vi "Scan Distributed Nodes.vi"(6 "ScanPeroid(>2000ms)":u32=2000, 8 "error in (no error)":errorcluster, 11 "Report Address":cluster{"address":string, "receiver port":u16}={"address"="234.5.6.7", "receiver port"=58432}) -> (0 "error out":errorcluster, 3 "Information":T1(array[cluster]))   [LabVIEW 2017]
doc: "Creates a read-only UDP multicast session and receives data on the specified port."
uses:
  _Typedef/Def-Report -- Cluster.ctl
  <vilib>/Utility/tcp.llb/UDP Multicast Read-Only Open.vi
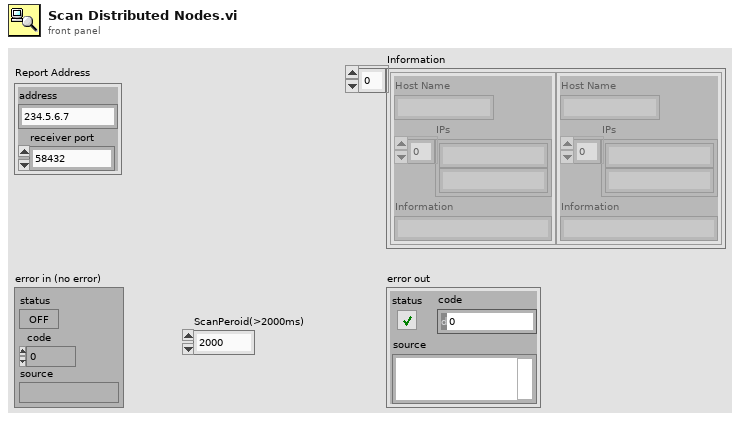
[diagram p1: front panel]
types:
  T1 = cluster{"Host Name":string, "IPs":string[], "Information":string}[]
  T2 = typedef "Def-Report -- Cluster.ctl" = cluster{"Host Name":string, "IPs":string[], "Timestamp":string, "Information":string}
  T3 = cluster{"Host Name":string, "IPs":string[], "Information":string}
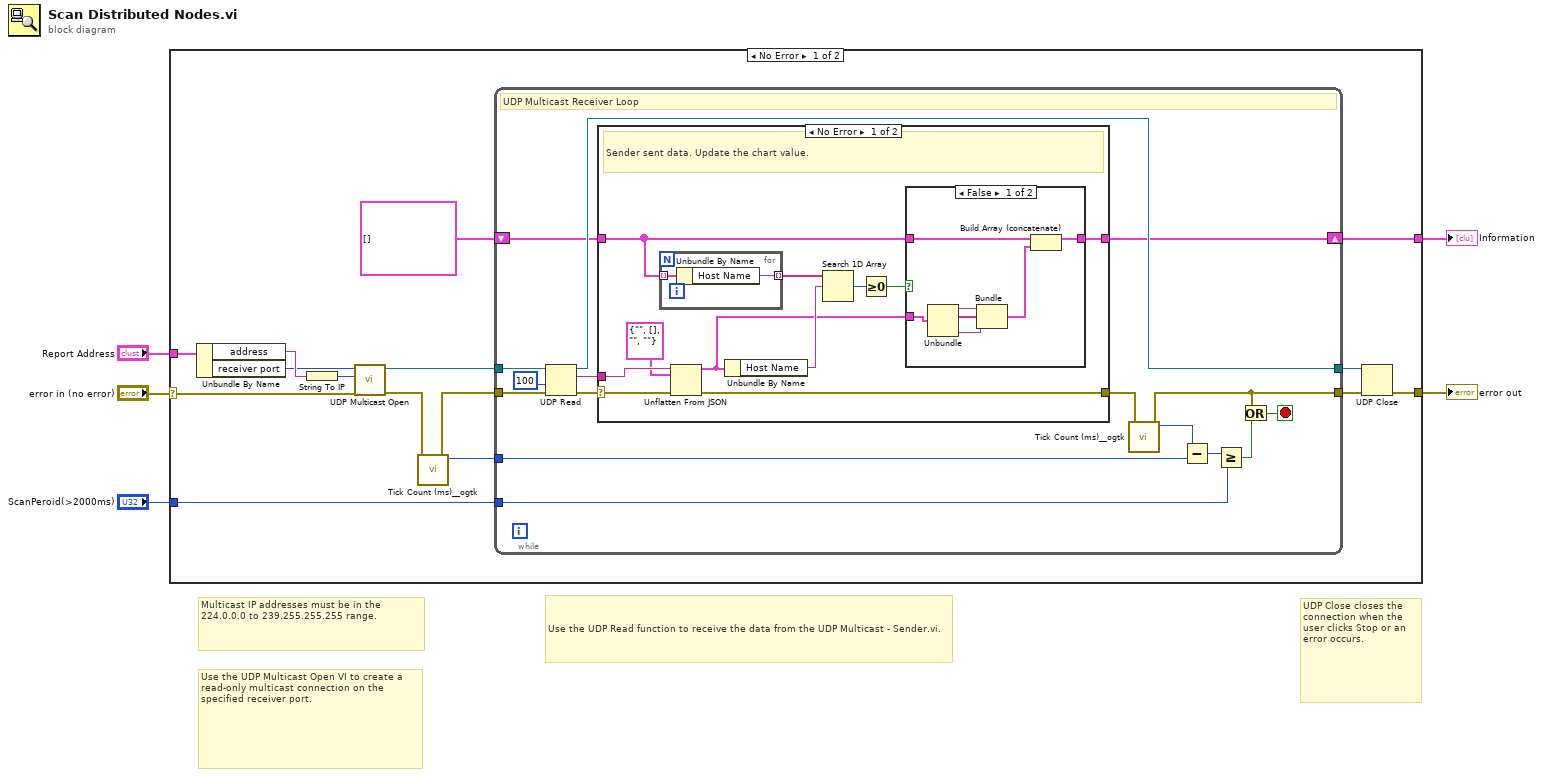
[diagram p0: block diagram]
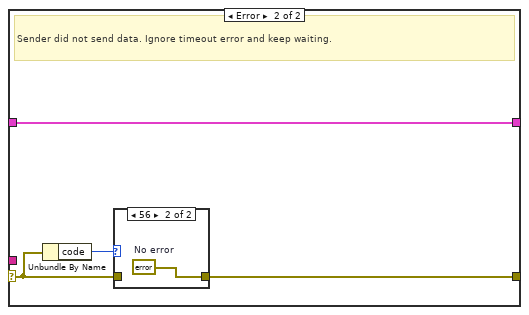
[diagram p3: hidden frame]
diagram:
  # "UDP Close closes the connection when the user clicks Stop or an error occurs."
  # "Use the UDP Multicast Open VI to create a read-only multicast connection on the specified receiver port."
  # "Multicast IP addresses must be in the 224.0.0.0 to 239.255.255.255 range."
  # "Use the UDP Read function to receive the data from the UDP Multicast - Sender.vi."
  n1 = case shown="No Error" "error in (no error)" {
    selector: "error in (no error)" -> [w12 w64]
    tunnel: "Report Address" -> [w15 _]
    tunnel: [w11 w64] -> w3
    tunnel: "ScanPeroid(>2000ms)" -> [w8 _]
    tunnel: [w6 _] -> w1
    frame No Error {
      n2 = Unbundle By Name(w15) -> ("address"=w14:string, "receiver port"=w13:u16)
      n3 = String To IP(1:w14) -> (0:w16:u32)
      n4 = call-poly <vilib>:"UDP Multicast Open.vi"("error in (no error)"=w12, "multicast addr"=w16, "port"=w13) -> ("error out"=w18:errorcluster, "connection ID"=w17:refnum<k16>)  [unwired: 6 in, 1 out]
      n5 = call <userlib>:"Tick Count (ms)__ogtk.vi"("error in (no error)"=w18) -> ("error out"=w10:errorcluster, "millisecond timer value"=w9:u32)  [unwired: 9 in]
      n6 = while {
        tunnel: w17 -> [w36]
        tunnel: [w29] -> w20
        tunnel: w10 -> [w34]
        tunnel: [w21] -> w19
        tunnel: w9 -> [w27]
        tunnel: w8 -> [w25]
        shift-right: [w22] -> w6
        shift-left: T1 [] ("Pack") -> [w23]
        stop <- w35 stop-if-true
        # "UDP Multicast Receiver Loop"
        n7 = UDP Read(connection ID=w36, timeout ms (25000)=100, 8:w34) -> (data out=w32:string, error out=w31:errorcluster, 3:w29:refnum<k16>)  [unwired: 3 out]
        n8 = case shown="No Error" w31 {
          selector: w31 -> [w47 w60]
          tunnel: w32 -> [w45 _]
          tunnel: [w46 w59] -> w30
          tunnel: w23 -> [w38 w58]
          tunnel: [w39 w58] -> w22
          frame No Error {
            # "Sender sent data. Update the chart value."
            n9 = for {
              tunnel: w38 -> [w57] mode=indexing
              tunnel: [w56] -> w43 mode=indexing
              n10 = Unbundle By Name(w57) -> ("Host Name"=w56:string)
            }
            n11 = Unflatten From JSON(JSON string=w45, type and defaults=T2 {"Host Name"="", "IPs"=[], "Timestamp"="", "Information"=""} ("Pack"), error in (no error)=w47) -> (value=w37:T2, error out=w46:errorcluster)  [unwired: 4 in]
            n12 = Unbundle By Name(w37) -> ("Host Name"=w42:string)
            n13 = Search 1D Array(1D array=w43, element=w42) -> (index of element=w41:i32)  [unwired: 1 in]
            n14 = Greater Or Equal To 0?(x=w41) -> (x >= 0?=w40:bool)
            n15 = case shown="False" w40 {
              tunnel: [w53 w55] -> w39
              tunnel: w38 -> [w54 w55]
              tunnel: w37 -> [w52 _]
              frame False {
                n16 = Unbundle(w52) -> ("Host Name"=w51:string, "IPs"=w50:string[], "Information"=w48:string)  [unwired: 1 out]
                n17 = Bundle("Host Name"=w51, "IPs"=w50, "Information"=w48) -> (w49:T3)  [unwired: 1 in]
                n18 = Build Array (concatenate)(w54, w49) -> (w53:T1)
              }
              frame True {
              }
            }
          }
          frame Error {
            # "Sender did not send data. Ignore timeout error and keep waiting."
            n19 = Unbundle By Name(w60) -> ("code"=w61:i32)
            n20 = case shown="56" w61 {
              tunnel: w60 -> [w62 _]
              tunnel: [w62 w63] -> w59
              frame Default {
              }
              frame 56 {
                w63 = errorcluster {"status"=FALSE, "code"=0, "source"=""}  # No error
              }
            }
          }
        }
        n21 = call <userlib>:"Tick Count (ms)__ogtk.vi"("error in (no error)"=w30) -> ("error out"=w21:errorcluster, "millisecond timer value"=w28:u32)  [unwired: 9 in]
        n22 = Subtract(x=w28, y=w27) -> (x-y=w26:u32)
        n23 = Greater Or Equal?(x=w26, y=w25) -> (x >= y?=w24:bool)
        n24 = Or(x=w21, y=w24) -> (x .or. y?=w35:bool)
      }
      n25 = UDP Close(connection ID=w20, 8:w19) -> (error out=w11:errorcluster)  [unwired: 1 out]
    }
    frame Error {
    }
  }
  "error out" <- w3
  "Information" <- w1
